vi "FPGAController_v4.2.vi"() -> ()   [LabVIEW 2015]
uses:
  <vilib>/Utility/miscctls.llb/LVPointTypeDef.ctl
  <vilib>/FPGAPlugInAG/PXI-7954R/niLvFpga_Open_PXI-7954R.vi
  <userlib>/_OpenG.lib/file/file.llb/Strip Path Extension - Path__ogtk.vi
  <userlib>/_OpenG.lib/comparison/comparison.llb/DBL Changed__ogtk.vi
  <vilib>/Utility/error.llb/Error Cluster From Error Code.vi
  <vilib>/rvi/errors/niLvFpgaAdjustHostInterfaceError.vi
  <vilib>/addons/database/Connection.llb/Conn Execute.vi
  <vilib>/addons/database/Recordset.llb/Rec Fetch Recordset Data (R).vi
  <vilib>/addons/database/Recordset.llb/Rec Destroy - Connection.vi
  <vilib>/FPGAPlugInAG/PXI-7954R/niLvFpga_Close_PXI-7954R.vi
  <vilib>/rvi/interface/nirviOpenFPGA/nirviOpenFPGA.xnode
  FPGA Bitfiles/correlationwithf_FPGATarget_FPGAcode60214_dpdmgs7o1BA.lvbitx
  <vilib>/rvi/interface/nirviMethod/nirviMethod.xnode
  <vilib>/FPGA/interface/niFpgaViExecutionMode.ctl
  <vilib>/rvi/interface/nirviReadWriteControl/nirviReadWriteControl.xnode
  <vilib>/addons/database/_DB Variant To Data/Database Variant To Data.xnode
  <vilib>/rvi/interface/nirviCloseFPGA/nirviCloseFPGA.xnode
  <vilib>/addons/database/NI_Database_API.lvlib
  NiFpgaLv.dll
panel:
  in  "Tab Control":enum32{"Auto Threshold", "Manual Threshold"}(tab)
  in  "Refresh PSU":bool=TRUE
  in  "Auto Threshold":bool
  in  "Update All":bool
  in  "Raise Threshold":bool
  in  "Lower Threshold":bool
  in  "Threshold 1":bool
  in  "Threshold 2":bool
  in  "Threshold 3":bool
  in  "Threshold 4":bool
  in  "Threshold 5":bool
  in  "Threshold 6":bool
  in  "Threshold 7":bool
  in  "Update By":i32
  out "Time Betwee Shots":dbl
  out "Del Armed":bool
  out "Update Threshold":bool
  in  "Min. Time\nBetween Shots (s)":dbl
  in  "Rate Limiting":bool
  out "Armed":bool
  in  "Add Delay":bool
  in  "Delay Name":string
  in  "Delay Value":dbl=3.0 min=0.0
  in  "Delay Ring":dbl(ring)=3.15039 items=["Custom"]
  in  "Rearm Trigger":bool
  in  "One Shot Mode":bool
  out "Last Update:":timestamp
  out "Updating FPGA":bool
  out "Sensitivity":dbl
  out "error out":errorcluster
  out "Low Mass Limit":fxp<+,31,17>
  out "High Mass Limit":fxp<+,31,17>
  out "stopping":bool
  out "Peletron (MV)":dbl=2.0
  out "High Mass (kg)":dbl=inf
  out "Low Mass (kg)":dbl
  out "High Charge Limit":i16
  out "Low Charge Limit":i16
  out "High velocity count":i32=210
  out "Low velocity count":i32=21000
  in  "stop":bool
  in  "Peak-Threshold Factor":dbl=2.0
  out "Low Charge Limit (fC)":dbl
  out "High Charge Limit (fC)":dbl=100.0
  out "High Velocity":dbl=100000.0
  out "Low Velocity":dbl=1000.0
  out "Filter 7 Peak":i32=7483
  out "Filter 6 Peak":i32=9863
  out "Filter 5 Peak":i32=13910
  out "Filter 4 Peak":i32=18191
  out "Filter 3 Peak":i32=46254
  out "Filter 2 Peak":i32=120664
  out "Filter 1 Peak":i32=295996
  in  "Filter7 Threshold":i32=-21165
  in  "Filter6 Threshold":i32=-29358
  in  "Filter5 Threshold":i32=-41730
  in  "Filter4 Threshold":i32=-54306
  in  "Filter3 Threshold":i32=-138762
  in  "Filter2 Threshold":i32=-361992
  in  "Filter1 Threshold":i32=-887988
  in  "Zero Peak Values":bool
  in  "Assign Threshold":bool
  in  "Run Mode":bool
  # "Settings"
  # "Dubugging"
  # "Independent Variable"
  # "Low Vel."
  # "High Vel."
  # "Low Q (fC)"
  # "High Q (fC)"
  # "Plate Control While Loop Counter"
  # "Low Mass (kg)"
  # "High Mass (kg)"
  # "Sens. (V/pC)"
  # "Peletron (MV)"
  # "Current Value of Running Average"
  # "Peak Threshold Factor"
  # "Delay Trigger"
  # "Dist. from 2nd Det. (m)"
  # "Name"
  # "Peak Values"
  # "Peak 1"
  # "Peak 2"
  # "Peak 3"
  # "Peak 4"
  # "Peak 5"
  # "Peak 6"
  # "Peak 7"
  # "Thresholds"
  # "Threshold 1"
  # "Threshold 2"
  # "Threshold 3"
  # "Threshold 4"
  # "Threshold 5"
  # "Threshold 6"
  # "Threshold 7"
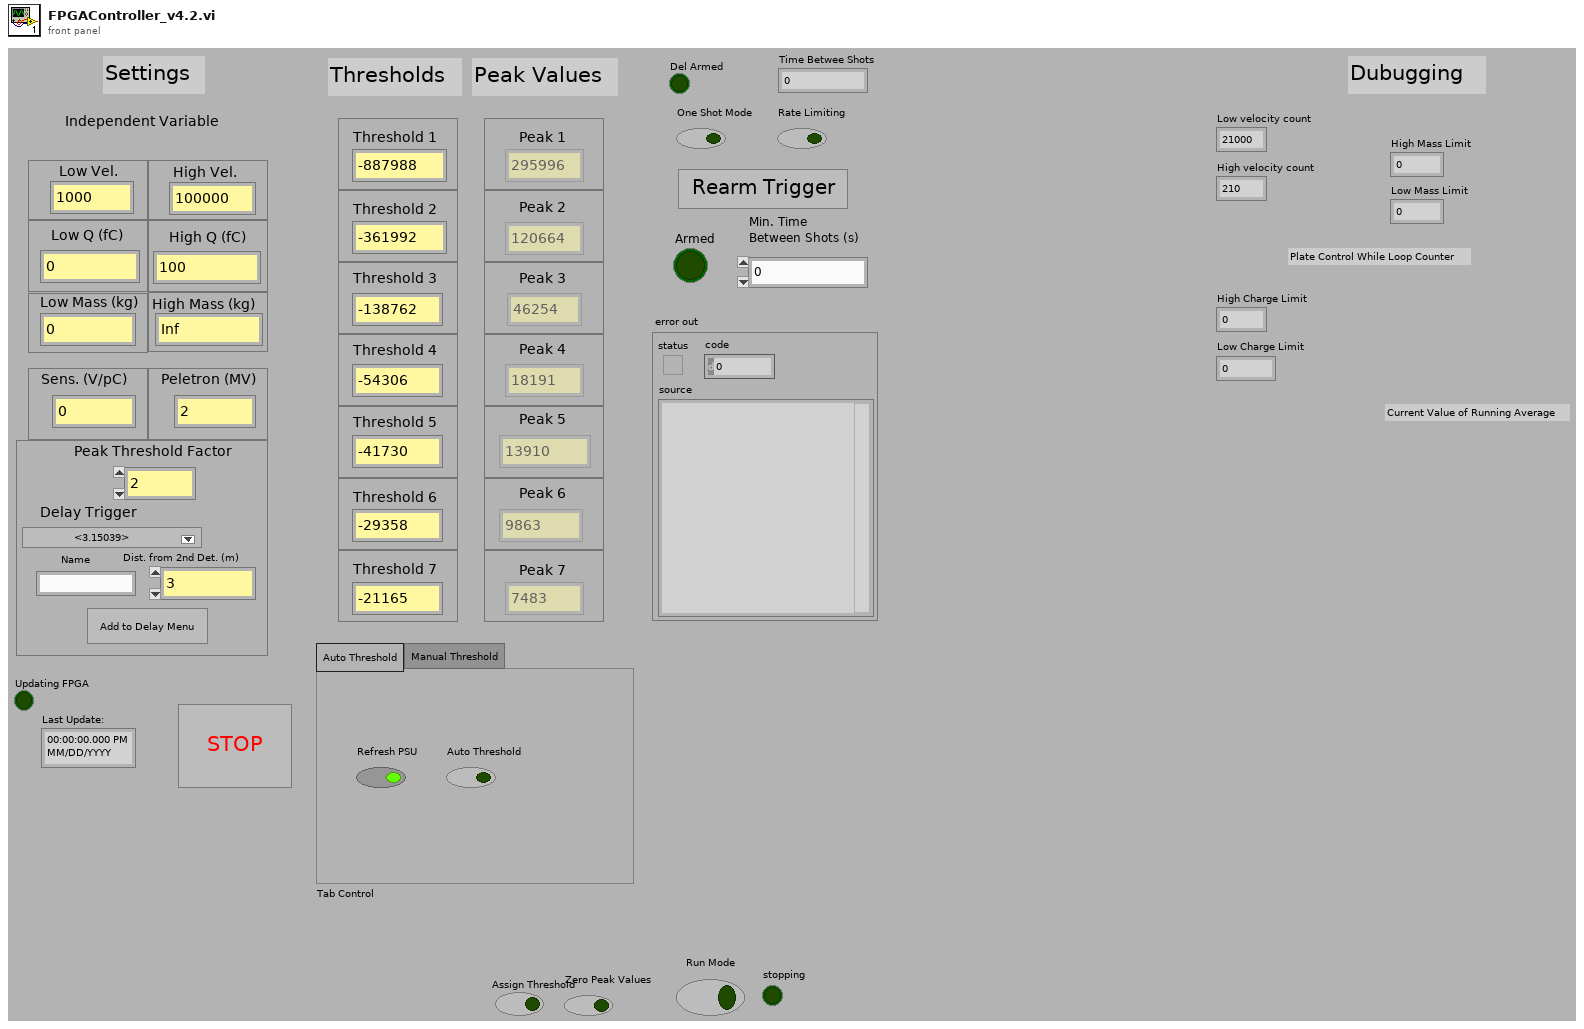
[diagram p1: front panel]
types:
  T1 = typedef "LVPointTypeDef.ctl" = cluster{"Horizontal":i16, "Vertical":i16}
  T2 = enum8{"Enabled", "Disabled", "Disabled and Grayed Out"}
  T3 = typedef "NI_Database_API.lvlib/Conn ObjectReference.ctl" = refnum<k1>
  T4 = typedef "NI_Database_API.lvlib/Rec ObjectReference.ctl" = refnum<k1>
  T5 = cluster{"Filter 1 Peak":i32, "Filter 2 Peak":i32, "Filter 3 Peak":i32, "Filter 4 Peak":i32, "Filter 5 Peak":i32, "Filter 6 Peak":i32, "Filter 7 Peak":i32}
  T6 = typedef "LVStringsAndValuesArrayTypeDef_DBL.ctl" = cluster{"String":string, "Value":dbl}[]
  T7 = cluster{"Numeric":dbl, "Numeric":dbl, "Numeric":dbl, "Numeric":dbl, "Numeric":dbl, "Numeric":dbl, "Sensitivity":dbl, dbl, "Value":dbl, fxp<+,16,7>, bool}
  T8 = cluster{"Low Velocity Count":i32, "High Velocity Count":i32, "Low Charge Limit (ADC ticks)":i16, "High Charge Limit (ADC ticks)":i16, "Low Mass (ADC*cycle^2)":i64, "High Mass (ADC*cycle^2)":i64, "Mult":fxp<+,16,7>, "Mult Use?":bool}
  T9 = cluster{"Filter 1 Detector 3 Correlation":i32, "Filter 2 Detector 3 Correlation":i32, "Filter 3 Detector 3 Correlation":i32, "Filter 4 Detector 3 Correlation":i32, "Filter 5 Detector 3 Correlation":i32, "Filter 6 Detector 3 Correlation":i32, "Filter 7 Detector 3 Correlation":i32}
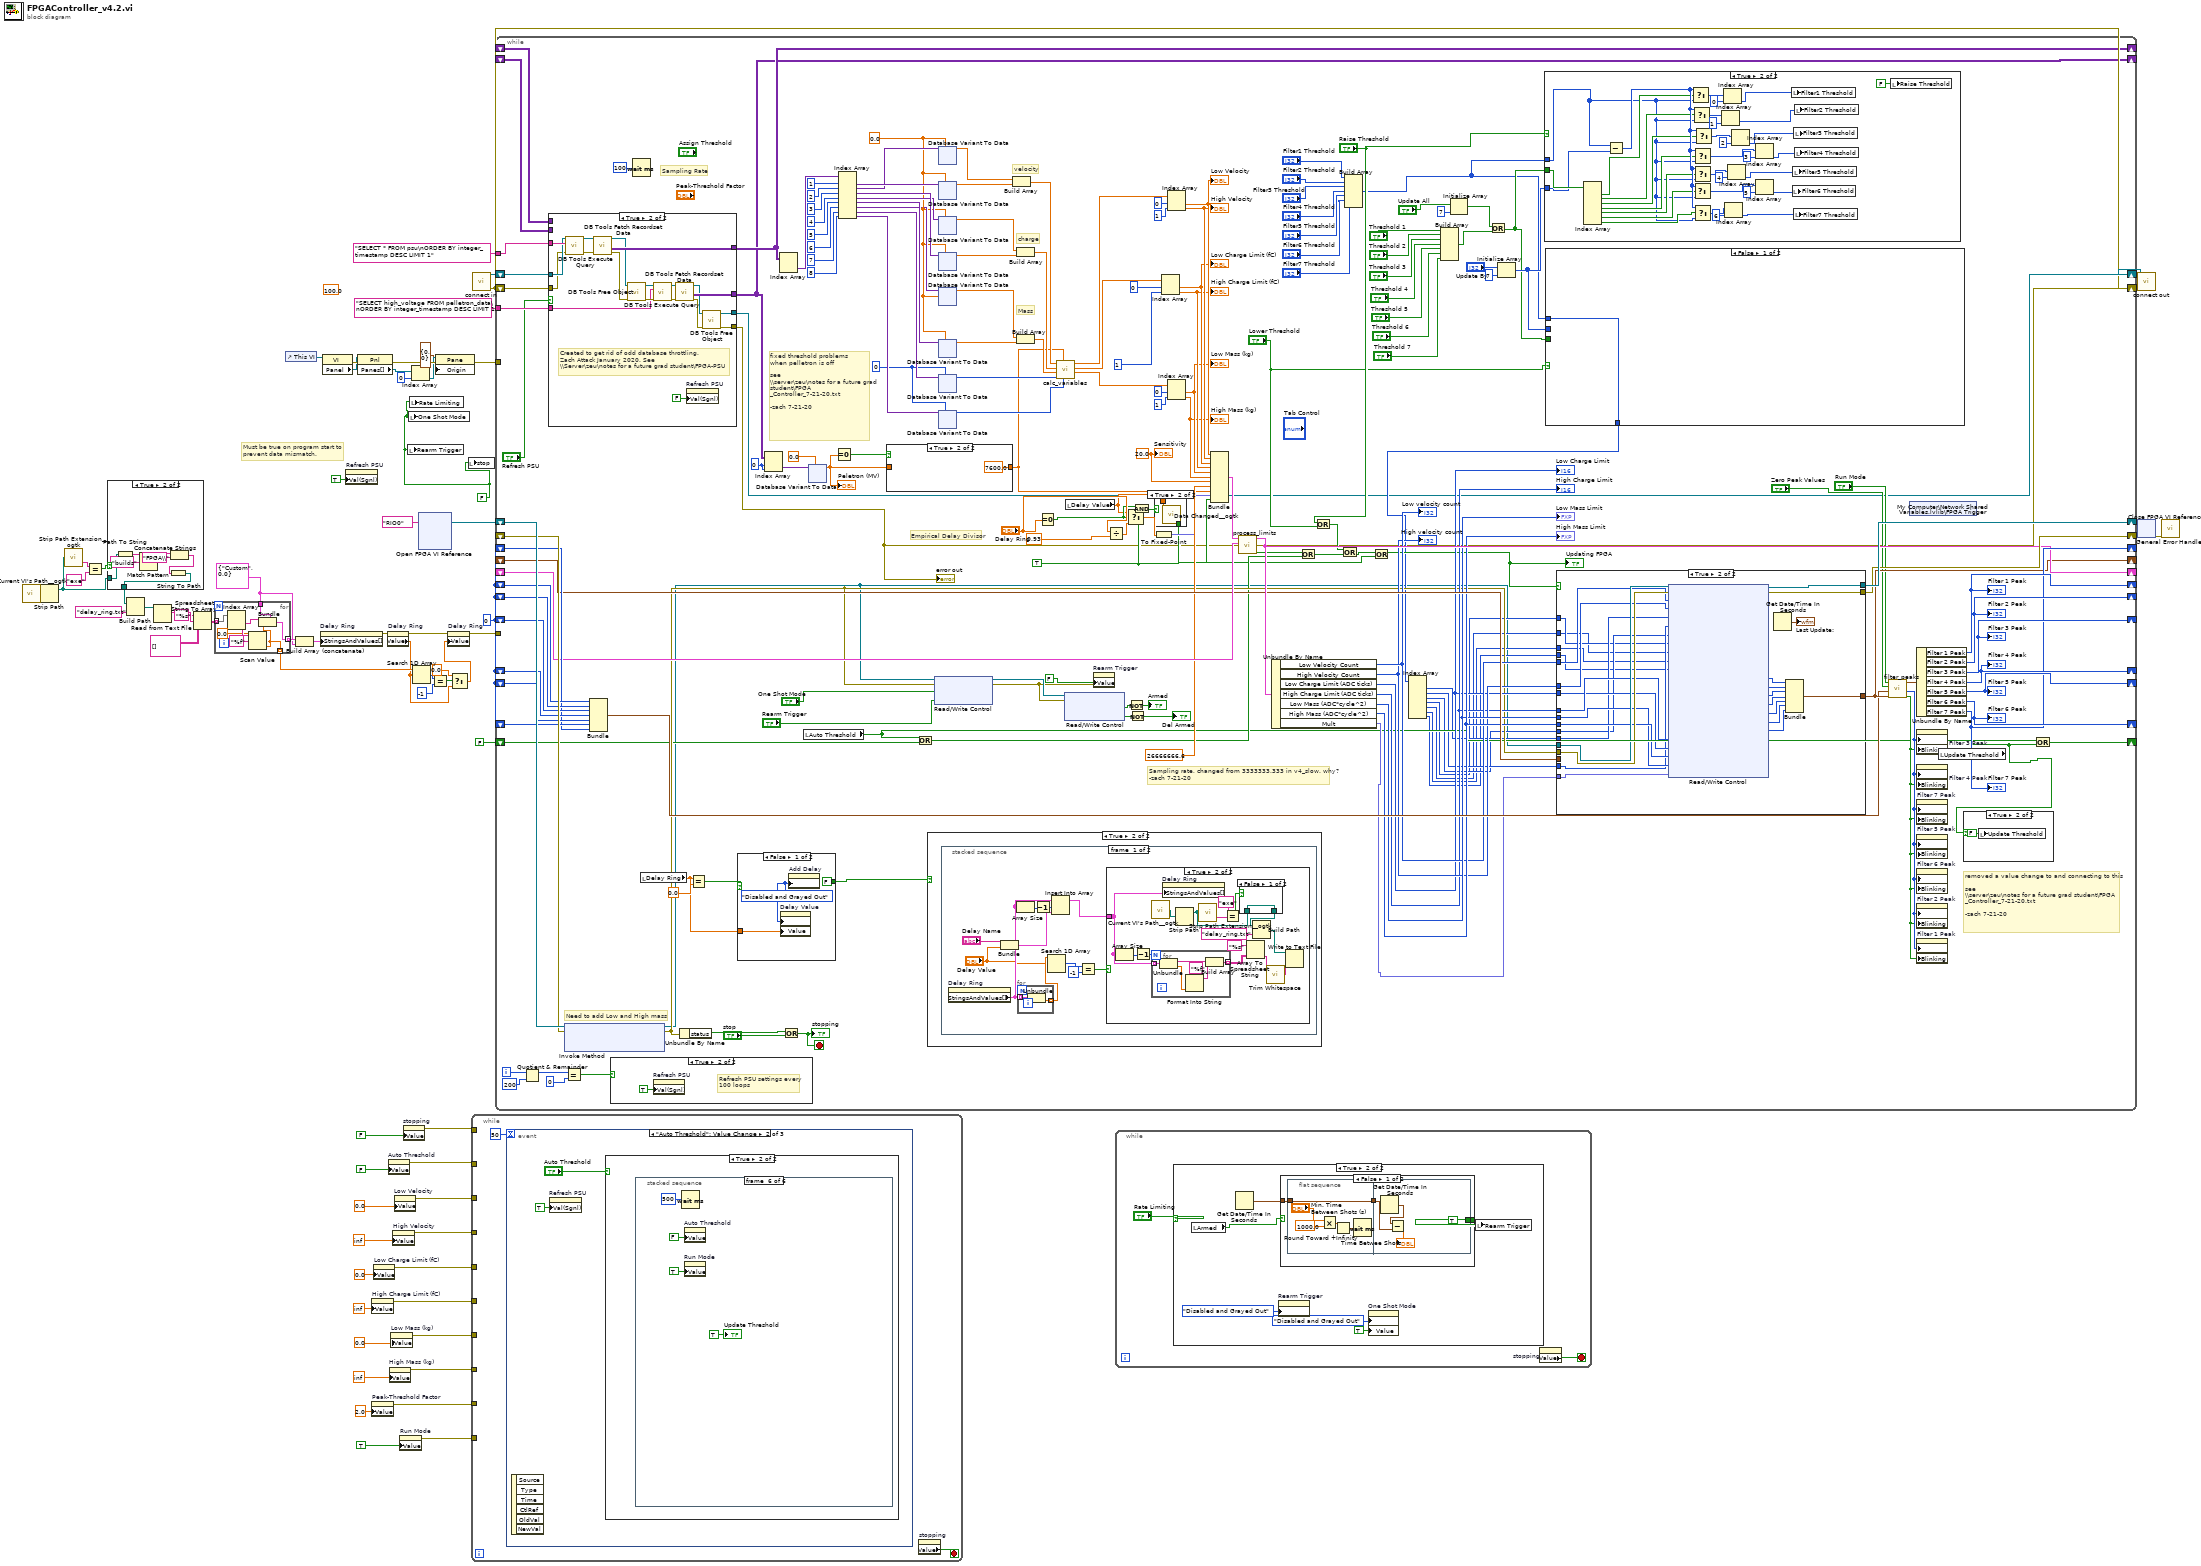
[diagram p0: block diagram]
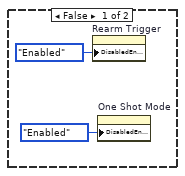
[diagram p3: hidden frame]
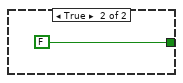
[diagram p4: hidden frame]
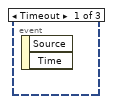
[diagram p5: hidden frame]
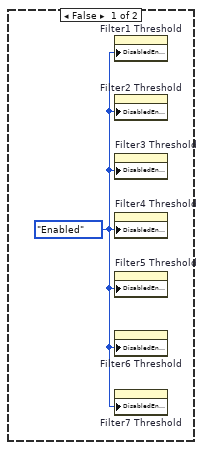
[diagram p6: hidden frame]
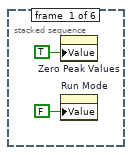
[diagram p7: hidden frame]
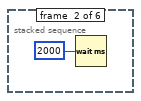
[diagram p8: hidden frame]
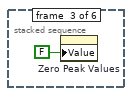
[diagram p9: hidden frame]
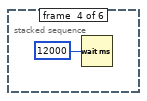
[diagram p10: hidden frame]
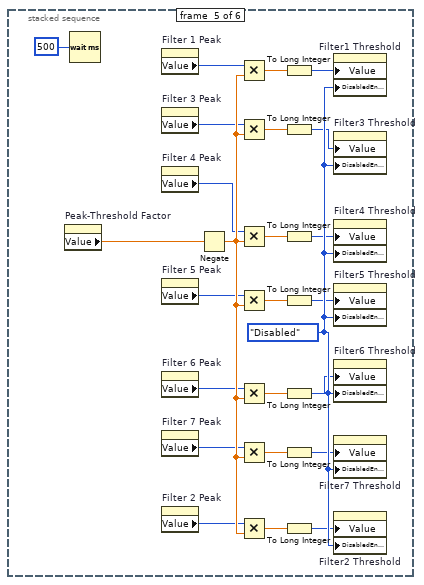
[diagram p11: hidden frame]
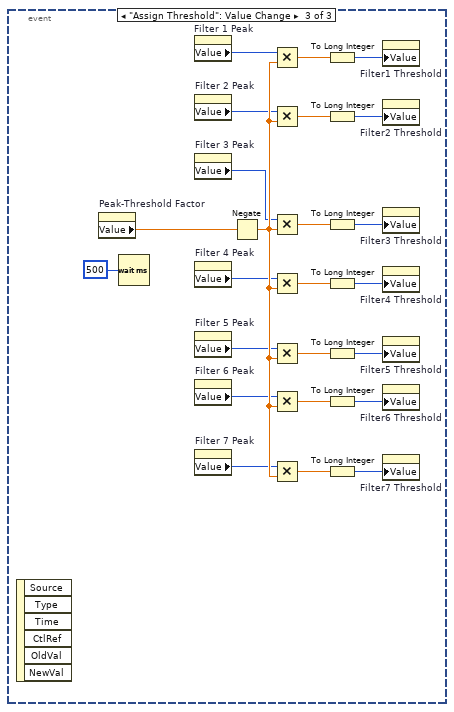
[diagram p12: hidden frame]
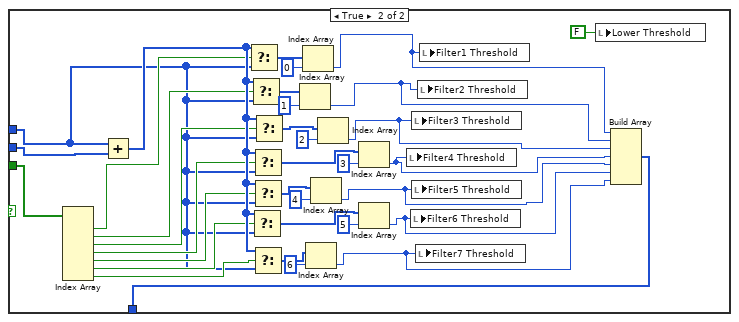
[diagram p16: hidden frame]
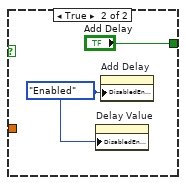
[diagram p20: hidden frame]
diagram:
  (unwired) 100.0 ("Update By")
  w19 = cluster{"String":string, "Value":dbl} {"String"="Custom", "Value"=0.0}
  w29 = FALSE
  w67 = 0
  # "Must be true on program start to\nprevent data mismatch."
  n1 = call <userlib>:"Current VI's Path__ogtk.vi"() -> ("Current VI's Path (+ Relative)"=w28:path)  [unwired: 1 in]
  n2 = Strip Path(path=w28) -> (stripped path=w14:path)  [unwired: 1 out]
  n3 = call-poly <userlib>:"Strip Path Extension__ogtk.vi"("path"=w14) -> ("extension"=w18:string)  [unwired: 1 out]
  n4 = Equal?(x=w18, y="exe") -> (x = y?=w15:bool)
  n5 = case shown="True" w15 {
    tunnel: w14 -> [w69 w76]
    tunnel: [w69 w70] -> w13
    frame False {
    }
    frame True {
      n6 = Path To String(path=w76) -> (string=w75:string)
      n7 = Match Pattern(string=w75, regular expression="builds") -> (before substring=w73:string)  [unwired: 1 in, 3 out]
      n8 = Concatenate Strings(w73, "FPGA\\" ("string")) -> (w71:string)
      n9 = String To Path(string=w71) -> (path=w70:path)
    }
  }
  n10 = Build Path(base path=w13, name or relative path="delay_ring.txt") -> (appended path=w16:path)
  n11 = Read from Text File(file (use dialog)=w16) -> (text=w26:string)  [unwired: 3 in, 3 out]
  n12 = Spreadsheet String To Array(format string="%s", spreadsheet string=w26, array type (2D Dbl)=string[][] []) -> (array=w23:string[][])  [unwired: 1 in]
  n13 = for {
    tunnel: w23 -> [w84] mode=indexing
    tunnel: w19 -> [w82]
    tunnel: [w78] -> w20 mode=indexing
    tunnel: [w77] -> w12 mode=indexing
    n14 = Index Array(array=w84) -> (element #1=w83:string, element #2=w81:string)  [unwired: 2 in]
    n15 = Scan Value(string=w81, format string="%f", default (0 dbl)=0.0) -> (value=w77:dbl)  [unwired: 1 out]
    n16 = Bundle(cluster=w82, "String"=w83, "Value"=w77) -> (w78:cluster{"String":string, "Value":dbl})
  }
  n17 = control-ref of="This VI"() -> (w40:refnum<vi>)
  n18 = Build Array (concatenate)(w20, w19) -> (w22:cluster{"String":string, "Value":dbl}[])
  n19 = property on="Delay Ring" class="Ring (strict)"("StringsAndValues[]"=w22) -> (error out=w21:errorcluster)  [unwired: 2 in, 1 out]
  n20 = property class="VI"(reference=w40) -> (error out=w39:errorcluster, "Panel"=w38:refnum<vi>)  [unwired: 1 in, 1 out]
  n21 = property on="Refresh PSU" class="Bool (strict)"("Val(Sgnl)"=TRUE ("Value (Signaling)")) -> ()  [unwired: 2 in, 2 out]
  n22 = property class="Pnl"(reference=w38, error in=w39) -> (error out=w37:errorcluster, "Panes[]"=w36:refnum<vi>[])  [unwired: 1 out]
  n23 = property on="High Charge Limit (fC)" class="DigNum (strict)"("Value"=inf ("High Charge Limit (fC)")) -> (error out=w54:errorcluster)  [unwired: 2 in, 1 out]
  n24 = property on="Peak-Threshold Factor" class="DigNum (strict)"("Value"=2.0 ("Peak-Threshold Factor")) -> (error out=w48:errorcluster)  [unwired: 2 in, 1 out]
  n25 = property on="Low Charge Limit (fC)" class="DigNum (strict)"("Value"=0.0 ("Low Charge Limit (fC)")) -> (error out=w56:errorcluster)  [unwired: 2 in, 1 out]
  n26 = property on="Delay Ring" class="Ring (strict)"(error in=w21) -> (error out=w11:errorcluster, "Value"=w5:dbl)  [unwired: 1 in, 1 out]
  n27 = property on="Auto Threshold" class="Bool (strict)"("Value"=FALSE ("Auto Threshold")) -> (error out=w62:errorcluster)  [unwired: 2 in, 1 out]
  n28 = property on="High Mass (kg)" class="DigNum (strict)"("Value"=inf ("High Mass (kg)")) -> (error out=w50:errorcluster)  [unwired: 2 in, 1 out]
  n29 = property on="Low Mass (kg)" class="DigNum (strict)"("Value"=0.0 ("Low Mass (kg)")) -> (error out=w52:errorcluster)  [unwired: 2 in, 1 out]
  n30 = property on="High Velocity" class="DigNum (strict)"("Value"=inf ("High Velocity")) -> (error out=w58:errorcluster)  [unwired: 2 in, 1 out]
  n31 = property on="Low Velocity" class="DigNum (strict)"("Value"=0.0 ("Low Velocity")) -> (error out=w60:errorcluster)  [unwired: 2 in, 1 out]
  n32 = property on="Run Mode" class="Bool (strict)"("Value"=TRUE ("Run Mode")) -> (error out=w46:errorcluster)  [unwired: 2 in, 1 out]
  n33 = property on="stopping" class="Bool (strict)"("Value"=FALSE ("stopping")) -> (error out=w64:errorcluster)  [unwired: 2 in, 1 out]
  n34 = local write "Rearm Trigger"(w29) -> ()
  n35 = local write "One Shot Mode"(w29) -> ()
  n36 = local write "Rate Limiting"(w29) -> ()
  n37 = Index Array(array=w36, index=0) -> (element=w34:refnum<vi>)
  n38 = Search 1D Array(1D array=w12, element=w5) -> (index of element=w9:i32)  [unwired: 1 in]
  n39 = xnode "Open FPGA VI Reference"("resource name"=tag "RIO0") -> ("FPGA VI Reference Out"=w31:refnum<k20>)  [unwired: 1 in, 1 out]
  n40 = Equal?(x=w9, y=-1) -> (x = y?=w7:bool)
  n41 = property class="Pane"(reference=w34, error in=w37, "Origin"=T1 {"Horizontal"=0, "Vertical"=0}) -> (error out=w32:errorcluster)  [unwired: 1 out]
  n42 = Select(t=0.0, s=w7, f=w5) -> (s? t:f=w6:dbl)
  n43 = property on="Delay Ring" class="Ring (strict)"(error in=w11, "Value"=w6) -> (error out=w10:errorcluster)  [unwired: 1 in, 1 out]
  n44 = local write "stop"(w29) -> ()
  n45 = while {
    tunnel: w64 -> [_]
    tunnel: w62 -> [_]
    tunnel: w60 -> [_]
    tunnel: w58 -> [_]
    tunnel: w56 -> [_]
    tunnel: w54 -> [_]
    tunnel: w52 -> [_]
    tunnel: w50 -> [_]
    tunnel: w48 -> [_]
    tunnel: w46 -> [_]
    stop <- w86 stop-if-true
    n46 = event shown="[1] \"Auto Threshold\": Value Change" {
      selector: _ -> [_ _ _]
      dyn-events: _ -> [_ _ _]
      timeout: 50 -> [_ _ _]
      event Timeout {
        n47 = event-data() -> ()  [unwired: 1 in, 2 out]
      }
      event "Auto Threshold": Value Change {
        n48 = event-data() -> ()  [unwired: 1 in, 6 out]
        n49 = property on="Refresh PSU" class="Bool (strict)"("Val(Sgnl)"=TRUE ("Value (Signaling)")) -> ()  [unwired: 2 in, 2 out]
        n50 = case shown="True" "Auto Threshold" {
          frame False {
            w89 = T2."Enabled" ("Disabled")
            n51 = property on="Filter1 Threshold" class="DigNum (strict)"("DisabledEnum"=w89) -> ()  [unwired: 2 in, 2 out]
            n52 = property on="Filter2 Threshold" class="DigNum (strict)"("DisabledEnum"=w89) -> ()  [unwired: 2 in, 2 out]
            n53 = property on="Filter3 Threshold" class="DigNum (strict)"("DisabledEnum"=w89) -> ()  [unwired: 2 in, 2 out]
            n54 = property on="Filter4 Threshold" class="DigNum (strict)"("DisabledEnum"=w89) -> ()  [unwired: 2 in, 2 out]
            n55 = property on="Filter5 Threshold" class="DigNum (strict)"("DisabledEnum"=w89) -> ()  [unwired: 2 in, 2 out]
            n56 = property on="Filter6 Threshold" class="DigNum (strict)"("DisabledEnum"=w89) -> ()  [unwired: 2 in, 2 out]
            n57 = property on="Filter7 Threshold" class="DigNum (strict)"("DisabledEnum"=w89) -> ()  [unwired: 2 in, 2 out]
          }
          frame True {
            n58 = stacked-sequence {
              frame #0 {
                n59 = property on="Zero Peak Values" class="Bool (strict)"("Value"=TRUE ("Zero Peak Values")) -> ()  [unwired: 2 in, 2 out]
                n60 = property on="Run Mode" class="Bool (strict)"("Value"=FALSE ("Run Mode")) -> ()  [unwired: 2 in, 2 out]
              }
              frame #1 {
                n61 = Wait (ms)(milliseconds to wait=u32 2000) -> ()  [unwired: 1 out]
              }
              frame #2 {
                n62 = property on="Zero Peak Values" class="Bool (strict)"("Value"=FALSE ("Zero Peak Values")) -> ()  [unwired: 2 in, 2 out]
              }
              frame #3 {
                n63 = Wait (ms)(milliseconds to wait=u32 12000) -> ()  [unwired: 1 out]
              }
              frame #4 {
                w119 = T2."Disabled" ("Disabled")
                n64 = property on="Peak-Threshold Factor" class="DigNum (strict)"() -> ("Value"=w104:dbl)  [unwired: 2 in, 2 out]
                n65 = Wait (ms)(milliseconds to wait=u32 500) -> ()  [unwired: 1 out]
                n66 = property on="Filter 1 Peak" class="DigNum (strict)"() -> ("Value"=w102:i32)  [unwired: 2 in, 2 out]
                n67 = property on="Filter 3 Peak" class="DigNum (strict)"() -> ("Value"=w100:i32)  [unwired: 2 in, 2 out]
                n68 = property on="Filter 4 Peak" class="DigNum (strict)"() -> ("Value"=w99:i32)  [unwired: 2 in, 2 out]
                n69 = property on="Filter 5 Peak" class="DigNum (strict)"() -> ("Value"=w98:i32)  [unwired: 2 in, 2 out]
                n70 = property on="Filter 6 Peak" class="DigNum (strict)"() -> ("Value"=w97:i32)  [unwired: 2 in, 2 out]
                n71 = property on="Filter 7 Peak" class="DigNum (strict)"() -> ("Value"=w96:i32)  [unwired: 2 in, 2 out]
                n72 = property on="Filter 2 Peak" class="DigNum (strict)"() -> ("Value"=w101:i32)  [unwired: 2 in, 2 out]
                n73 = Negate(x=w104) -> (-x=w103:dbl)
                n74 = Multiply(x=w102, y=w103) -> (x*y=w118:dbl)
                n75 = Multiply(x=w100, y=w103) -> (x*y=w114:dbl)
                n76 = Multiply(x=w99, y=w103) -> (x*y=w112:dbl)
                n77 = Multiply(x=w98, y=w103) -> (x*y=w110:dbl)
                n78 = Multiply(x=w97, y=w103) -> (x*y=w108:dbl)
                n79 = Multiply(x=w96, y=w103) -> (x*y=w106:dbl)
                n80 = Multiply(x=w101, y=w103) -> (x*y=w116:dbl)
                n81 = To Long Integer(number=w118) -> (32bit integer=w117:i32)
                n82 = To Long Integer(number=w114) -> (32bit integer=w113:i32)
                n83 = To Long Integer(number=w112) -> (32bit integer=w111:i32)
                n84 = To Long Integer(number=w110) -> (32bit integer=w109:i32)
                n85 = To Long Integer(number=w108) -> (32bit integer=w107:i32)
                n86 = To Long Integer(number=w106) -> (32bit integer=w105:i32)
                n87 = To Long Integer(number=w116) -> (32bit integer=w115:i32)
                n88 = property on="Filter1 Threshold" class="DigNum (strict)"("Value"=w117, "DisabledEnum"=w119) -> ()  [unwired: 2 in, 2 out]
                n89 = property on="Filter3 Threshold" class="DigNum (strict)"("Value"=w113, "DisabledEnum"=w119) -> ()  [unwired: 2 in, 2 out]
                n90 = property on="Filter4 Threshold" class="DigNum (strict)"("Value"=w111, "DisabledEnum"=w119) -> ()  [unwired: 2 in, 2 out]
                n91 = property on="Filter5 Threshold" class="DigNum (strict)"("Value"=w109, "DisabledEnum"=w119) -> ()  [unwired: 2 in, 2 out]
                n92 = property on="Filter6 Threshold" class="DigNum (strict)"("Value"=w107, "DisabledEnum"=w119) -> ()  [unwired: 2 in, 2 out]
                n93 = property on="Filter7 Threshold" class="DigNum (strict)"("Value"=w105, "DisabledEnum"=w119) -> ()  [unwired: 2 in, 2 out]
                n94 = property on="Filter2 Threshold" class="DigNum (strict)"("Value"=w115, "DisabledEnum"=w119) -> ()  [unwired: 2 in, 2 out]
              }
              frame #5 {
                n95 = Wait (ms)(milliseconds to wait=u32 500) -> ()  [unwired: 1 out]
                n96 = property on="Auto Threshold" class="Bool (strict)"("Value"=FALSE ("Auto Threshold")) -> ()  [unwired: 2 in, 2 out]
                n97 = property on="Run Mode" class="Bool (strict)"("Value"=TRUE ("Run Mode")) -> ()  [unwired: 2 in, 2 out]
                "Update Threshold" <- TRUE ("Update Threshold")
              }
            }
          }
        }
      }
      event "Assign Threshold": Value Change {
        n98 = event-data() -> ()  [unwired: 1 in, 6 out]
        n99 = property on="Peak-Threshold Factor" class="DigNum (strict)"() -> ("Value"=w138:dbl)  [unwired: 2 in, 2 out]
        n100 = Wait (ms)(milliseconds to wait=u32 500) -> ()  [unwired: 1 out]
        n101 = property on="Filter 1 Peak" class="DigNum (strict)"() -> ("Value"=w137:i32)  [unwired: 2 in, 2 out]
        n102 = property on="Filter 2 Peak" class="DigNum (strict)"() -> ("Value"=w136:i32)  [unwired: 2 in, 2 out]
        n103 = property on="Filter 3 Peak" class="DigNum (strict)"() -> ("Value"=w135:i32)  [unwired: 2 in, 2 out]
        n104 = property on="Filter 4 Peak" class="DigNum (strict)"() -> ("Value"=w134:i32)  [unwired: 2 in, 2 out]
        n105 = property on="Filter 5 Peak" class="DigNum (strict)"() -> ("Value"=w133:i32)  [unwired: 2 in, 2 out]
        n106 = property on="Filter 6 Peak" class="DigNum (strict)"() -> ("Value"=w132:i32)  [unwired: 2 in, 2 out]
        n107 = property on="Filter 7 Peak" class="DigNum (strict)"() -> ("Value"=w131:i32)  [unwired: 2 in, 2 out]
        n108 = Negate(x=w138) -> (-x=w140:dbl)
        n109 = Multiply(x=w137, y=w140) -> (x*y=w147:dbl)
        n110 = Multiply(x=w136, y=w140) -> (x*y=w145:dbl)
        n111 = Multiply(x=w135, y=w140) -> (x*y=w144:dbl)
        n112 = Multiply(x=w134, y=w140) -> (x*y=w143:dbl)
        n113 = Multiply(x=w133, y=w140) -> (x*y=w142:dbl)
        n114 = Multiply(x=w132, y=w140) -> (x*y=w141:dbl)
        n115 = Multiply(x=w131, y=w140) -> (x*y=w146:dbl)
        n116 = To Long Integer(number=w147) -> (32bit integer=w130:i32)
        n117 = To Long Integer(number=w145) -> (32bit integer=w129:i32)
        n118 = To Long Integer(number=w144) -> (32bit integer=w128:i32)
        n119 = To Long Integer(number=w143) -> (32bit integer=w127:i32)
        n120 = To Long Integer(number=w142) -> (32bit integer=w126:i32)
        n121 = To Long Integer(number=w141) -> (32bit integer=w125:i32)
        n122 = To Long Integer(number=w146) -> (32bit integer=w124:i32)
        n123 = property on="Filter1 Threshold" class="DigNum (strict)"("Value"=w130) -> ()  [unwired: 2 in, 2 out]
        n124 = property on="Filter2 Threshold" class="DigNum (strict)"("Value"=w129) -> ()  [unwired: 2 in, 2 out]
        n125 = property on="Filter3 Threshold" class="DigNum (strict)"("Value"=w128) -> ()  [unwired: 2 in, 2 out]
        n126 = property on="Filter4 Threshold" class="DigNum (strict)"("Value"=w127) -> ()  [unwired: 2 in, 2 out]
        n127 = property on="Filter5 Threshold" class="DigNum (strict)"("Value"=w126) -> ()  [unwired: 2 in, 2 out]
        n128 = property on="Filter6 Threshold" class="DigNum (strict)"("Value"=w125) -> ()  [unwired: 2 in, 2 out]
        n129 = property on="Filter7 Threshold" class="DigNum (strict)"("Value"=w124) -> ()  [unwired: 2 in, 2 out]
      }
    }
    n130 = property on="stopping" class="Bool (strict)"() -> ("Value"=w86:bool)  [unwired: 2 in, 2 out]
  }
  n131 = call "connect in.vi"() -> ("error out"=w41:errorcluster, "Database Connection"=w42:T3)  [unwired: 7 in, 1 out]
  n132 = while {
    shift-right: [w320] -> w66
    shift-left: w31 -> [w324]
    shift-right: [w319] -> w65
    shift-left: _ -> [w323]
    shift-right: [w315] -> _
    shift-left: w67 -> [w308]
    shift-right: [w314] -> _
    shift-left: w67 -> [w307]
    shift-right: [w313] -> _
    shift-left: w67 -> [w306]
    shift-right: [w312] -> _
    shift-left: w67 -> [w305]
    shift-right: [w311] -> _
    shift-left: w67 -> [w304]
    shift-right: [w317] -> _
    shift-left: w67 -> [w310]
    shift-right: [w316] -> _
    shift-left: w67 -> [w309]
    tunnel: "SELECT * FROM psu\nORDER BY integer_timestamp DESC LIMIT 1" ("SQL query") -> [w169]
    shift-right: [w165] -> w43
    shift-left: w42 -> [w168]
    shift-right: [w164] -> _
    shift-left: w41 -> [w167]
    shift-right: [w303] -> _
    shift-left: _ -> [w302]
    shift-right: [w300] -> _
    shift-left: _ -> [w301]
    tunnel: w32 -> [_]
    tunnel: w10 -> [_]
    shift-right: [w219] -> _
    shift-left: FALSE -> [w222]
    tunnel: "SELECT high_voltage FROM pelletron_data\nORDER BY integer_timestamp DESC LIMIT 1" ("SQL query") -> [w166]
    shift-right: [w163] -> _
    shift-left: _ -> [w162]
    shift-right: [w161] -> _
    shift-left: _ -> [w160]
    i -> [w158]
    stop <- w318 stop-if-true
    w151 = 20.0 ("Sensitivity")
    w191 = TRUE
    w266 = 0 ("index (row)")
    w267 = i8 0
    w268 = 0.0
    # "fixed threshold problems\nwhen pelletron is off\n\nsee \n\\\\server\\zeu\\notes for a future grad student\\FPGA\n_Controller_7-21-20.txt\n\n-zach 7-21-20"
    # "Sampling rate, changed from 3333333.333 in v4_slow. why?\n-zach 7-21-20"
    # "removed a value change to and connecting to this\n\nsee \n\\\\server\\zeu\\notes for a future grad student\\FPGA\n_Controller_7-21-20.txt\n\n-zach 7-21-20"
    # "charge"
    # "Empirical Delay Divisor"
    # "Mass"
    # "velocity"
    # "Sampling Rate"
    # "Need to add Low and High mass"
    n133 = Quotient & Remainder(x=w158, y=200) -> (x-y*floor(x/y)=w156:i32)  [unwired: 1 out]
    n134 = case shown="True" "Refresh PSU" {
      tunnel: [w329 w348] -> w163
      tunnel: w169 -> [_ w347]
      tunnel: w168 -> [w331 w346]
      tunnel: w167 -> [w330 w345]
      tunnel: w166 -> [_ w338]
      tunnel: [w328 w337] -> w161
      tunnel: [w331 w334] -> w165
      tunnel: [w330 w333] -> w164
      tunnel: w162 -> [w329 _]
      tunnel: w160 -> [w328 _]
      frame False {
      }
      frame True {
        # "Created to get rid of odd database throttling.\nZach Attack January 2020. See \n\\\\Server\\zeu\\notes for a future grad student\\FPGA-PSU"
        n135 = call-poly <vilib>:"DB Tools Execute Query.vi"("error in (no error)"=w345, "SQL query"=w347, "connection reference"=w346) -> ("error out"=w349:errorcluster, "recordset reference"=w350:T4)  [unwired: 5 in]
        n136 = call-poly <vilib>:"DB Tools Fetch Recordset Data.vi"("error in (no error)"=w349, "recordset reference"=w350) -> ("error out"=w339:errorcluster, "recordset data"=w348:variant[][], "recordset reference out"=w342:T4)  [unwired: 3 in]
        n137 = call-poly <vilib>:"DB Tools Free Object.vi"("error in (no error)"=w339, "recordset reference"=w342) -> ("error out"=w340:errorcluster, "connection reference"=w341:T3)  [unwired: 8 in]
        n138 = call-poly <vilib>:"DB Tools Execute Query.vi"("error in (no error)"=w340, "SQL query"=w338, "connection reference"=w341) -> ("error out"=w344:errorcluster, "recordset reference"=w343:T4)  [unwired: 5 in]
        n139 = call-poly <vilib>:"DB Tools Fetch Recordset Data.vi"("error in (no error)"=w344, "recordset reference"=w343) -> ("error out"=w335:errorcluster, "recordset data"=w337:variant[][], "recordset reference out"=w336:T4)  [unwired: 3 in]
        n140 = property on="Refresh PSU" class="Bool (strict)"("Val(Sgnl)"=FALSE ("Value (Signaling)")) -> ()  [unwired: 2 in, 2 out]
        n141 = call-poly <vilib>:"DB Tools Free Object.vi"("error in (no error)"=w335, "recordset reference"=w336) -> ("error out"=w333:errorcluster, "connection reference"=w334:T3)  [unwired: 8 in]
      }
    }
    "error out" <- w164
    n142 = xnode "Invoke Method"("FPGA VI Reference In"=w324, "error in"=w323) -> ("FPGA VI Reference Out"=w152:refnum<k20>, "error out"=w238:errorcluster)  [unwired: 1 out]
    n143 = Equal?(x=w156, y=0) -> (x = y?=w154:bool)
    n144 = Bundle("Filter 1 Peak"=w310, "Filter 2 Peak"=w309, "Filter 3 Peak"=w308, "Filter 4 Peak"=w307, "Filter 5 Peak"=w306, "Filter 6 Peak"=w305, "Filter 7 Peak"=w304) -> (w296:T5)  [unwired: 1 in]
    n145 = case shown="True" w154 {
      frame False {
      }
      frame True {
        # "Refresh PSU settings every\n100 loops"
        n146 = property on="Refresh PSU" class="Bool (strict)"("Val(Sgnl)"=TRUE ("Value (Signaling)")) -> ()  [unwired: 2 in, 2 out]
      }
    }
    n147 = Wait (ms)(milliseconds to wait=u32 100) -> ()  [unwired: 1 out]
    n148 = local read "Delay Ring"() -> (w223:dbl)
    n149 = Unbundle By Name(w238) -> ("status"=w322:bool)
    n150 = Equal?(x=w223, y=0.0) -> (x = y?=w224:bool)
    n151 = case shown="False" w224 {
      tunnel: [FALSE ("Add Delay") "Add Delay"] -> w241
      tunnel: w223 -> [w424 _]
      frame False {
        w425 = T2."Disabled and Grayed Out" ("Disabled")
        n152 = property on="Delay Value" class="DigNum (strict)"("DisabledEnum"=w425, "Value"=w424) -> ()  [unwired: 2 in, 2 out]
        n153 = property on="Add Delay" class="Bool (strict)"("DisabledEnum"=w425) -> ()  [unwired: 2 in, 2 out]
      }
      frame True {
        w426 = T2."Enabled" ("Disabled")
        n154 = property on="Delay Value" class="DigNum (strict)"("DisabledEnum"=w426) -> ()  [unwired: 2 in, 2 out]
        n155 = property on="Add Delay" class="Bool (strict)"("DisabledEnum"=w426) -> ()  [unwired: 2 in, 2 out]
      }
    }
    n156 = Index Array(array=w161, index (row)=w266, index (col)=w266) -> (element=w265:variant)
    n157 = Index Array(array=w163) -> (element=w277:variant[])  [unwired: 2 in]
    n158 = Or(x=w322, y="stop") -> (x .or. y?=w318:bool)
    "stopping" <- w318
    n159 = local read "Auto Threshold"() -> (w220:bool)
    n160 = xnode "Database Variant To Data"("database variant"=w265, "type"=0.0) -> ("data"=w149:dbl)  [unwired: 1 in, 1 out]
    "Peletron (MV)" <- w149
    n161 = Equal To 0?(x=w149) -> (x = 0?=w150:bool)
    n162 = Index Array(array=w277, index #1=1 ("index"), index #2=2 ("index"), index #3=3 ("index"), index #4=4 ("index"), index #5=5 ("index"), index #6=6 ("index"), index #7=7 ("index"), index #8=8 ("index")) -> (element #1=w276:variant, element #2=w275:variant, element #3=w274:variant, element #4=w273:variant, element #5=w272:variant, element #6=w271:variant, element #7=w270:variant, element #8=w269:variant)
    n163 = case shown="True" w150 {
      tunnel: [w325 7600.0 ("Value")] -> w148
      tunnel: w149 -> [w325 _]
      frame False {
      }
      frame True {
      }
    }
    n164 = Or(x=w220, y=w222) -> (x .or. y?=w221:bool)
    n165 = case shown="True" w241 {
      frame False {
      }
      frame True {
        n166 = stacked-sequence {
          frame #0 {
            n167 = property on="Delay Ring" class="Ring (strict)"() -> ("StringsAndValues[]"=w430:T6)  [unwired: 2 in, 2 out]
            n168 = Bundle("Delay Name"="Delay Name", "Delay Value"="Delay Value") -> (w435:cluster{"Delay Name":string, "Delay Value":dbl})  [unwired: 1 in]
            n169 = Array Size(array=w430) -> (size(s)=w433:i32)
            n170 = for {
              tunnel: w430 -> [w440] mode=indexing
              tunnel: [w439] -> w429 mode=indexing
              n171 = Unbundle(w440) -> ("Value"=w439:dbl)  [unwired: 1 out]
            }
            n172 = Decrement(x=w433) -> (x-1=w432:i32)
            n173 = Search 1D Array(1D array=w429, element="Delay Value") -> (index of element=w437:i32)  [unwired: 1 in]
            n174 = Insert Into Array(array=w430, index=w432, new element=w435) -> (w434:T6)
            n175 = Equal?(x=w437, y=-1) -> (x = y?=w431:bool)
            n176 = case shown="True" w431 {
              tunnel: w434 -> [_ w449]
              frame False {
                n177 = One Button Dialog(message="Value Already Exists") -> ()  [unwired: 1 in, 1 out]
              }
              frame True {
                n178 = Array Size(array=w449) -> (size(s)=w451:i32)
                n179 = Decrement(x=w451) -> (x-1=w450:i32)
                n180 = call <userlib>:"Current VI's Path__ogtk.vi"() -> ("Current VI's Path (+ Relative)"=w455:path)  [unwired: 1 in]
                n181 = for {
                  N: w450 -> [_]
                  tunnel: w449 -> [w465] mode=indexing
                  tunnel: [w460] -> w452 mode=indexing
                  n182 = Unbundle(w465) -> ("String"=w461:string, "Value"=w464:dbl)
                  n183 = Format Into String(format string="%f", w464) -> (resulting string=w462:string)  [unwired: 2 in, 1 out]
                  n184 = Build Array(w461, w462) -> (w460:string[])
                }
                n185 = property on="Delay Ring" class="Ring (strict)"("StringsAndValues[]"=w449) -> ()  [unwired: 2 in, 2 out]
                n186 = Strip Path(path=w455) -> (stripped path=w443:path)  [unwired: 1 out]
                n187 = call-poly <userlib>:"Strip Path Extension__ogtk.vi"("path"=w443) -> ("extension"=w446:string)  [unwired: 1 out]
                n188 = Equal?(x="exe", y=w446) -> (x = y?=w444:bool)
                n189 = case shown="False" w444 {
                  tunnel: w443 -> [w457 w459]
                  tunnel: [w457 w458] -> w442
                  frame False {
                  }
                  frame True {
                    n190 = Strip Path(path=w459) -> (stripped path=w458:path)  [unwired: 1 out]
                  }
                }
                n191 = Array To Spreadsheet String(array=w452, 3:"%s" ("format string")) -> (spreadsheet string=w448:string)  [unwired: 1 in]
                n192 = Build Path(base path=w442, name or relative path="delay_ring.txt") -> (appended path=w453:path)
                n193 = call <vilib>:"Trim Whitespace.vi"("string"=w448) -> ("trimmed string"=w447:string)  [unwired: 1 in]
                n194 = Write to Text File(file (use dialog)=w453, text=w447) -> ()  [unwired: 2 in, 3 out]
              }
            }
          }
          frame #1 {
            n195 = property on="Add Delay" class="Bool (strict)"("Value"=FALSE ("Add Delay")) -> ()  [unwired: 2 in, 2 out]
          }
        }
      }
    }
    n196 = xnode "Read/Write Control"("FPGA VI Reference In"=w152, "error in"=w238, "One Shot"="One Shot Mode", "Reset One Shot"="Rearm Trigger") -> ("FPGA VI Reference Out"=w232:refnum<k20>, "error out"=w231:errorcluster)
    n197 = xnode "Database Variant To Data"("database variant"=w275, "type"=w268) -> ("data"=w201:dbl)  [unwired: 1 in, 1 out]
    n198 = xnode "Database Variant To Data"("database variant"=w276, "type"=w268) -> ("data"=w202:dbl)  [unwired: 1 in, 1 out]
    n199 = xnode "Database Variant To Data"("database variant"=w273, "type"=w268) -> ("data"=w200:dbl)  [unwired: 1 in, 1 out]
    n200 = xnode "Database Variant To Data"("database variant"=w274, "type"=w268) -> ("data"=w199:dbl)  [unwired: 1 in, 1 out]
    n201 = xnode "Database Variant To Data"("database variant"=w271, "type"=w268) -> ("data"=w198:dbl)  [unwired: 1 in, 1 out]
    n202 = xnode "Database Variant To Data"("database variant"=w272, "type"=w268) -> ("data"=w197:dbl)  [unwired: 1 in, 1 out]
    n203 = xnode "Database Variant To Data"("database variant"=w270, "type"=w267) -> ("data"=w260:i8)  [unwired: 1 in, 1 out]
    n204 = xnode "Database Variant To Data"("database variant"=w269, "type"=w267) -> ("data"=w259:i8)  [unwired: 1 in, 1 out]
    n205 = Build Array(w201, w202) -> (w263:dbl[])
    n206 = Build Array(w200, w199) -> (w262:dbl[])
    n207 = Build Array(w198, w197) -> (w261:dbl[])
    n208 = Equal To 0?(x="Delay Ring") -> (x = 0?=w196:bool)
    n209 = call "calc_variables.vi"("var2"=w259, "Peletron"=w148, "var1"=w260, "Mass"=w261, "Charge"=w262, "Velocity"=w263) -> ("Mass out"=w252:dbl[], "Charge out"=w255:dbl[], "Velocity out"=w258:dbl[])  [unwired: 3 in]
    n210 = xnode "Read/Write Control"("FPGA VI Reference In"=w232, "error in"=w231) -> ("Not Armed?"=w230:bool, "Del Not Armed?"=w190:bool)  [unwired: 2 out]
    n211 = local read "Delay Value"() -> (w195:dbl)
    n212 = property on="Rearm Trigger" class="Bool (strict)"(error in=w231, "Value"=FALSE ("Rearm Trigger")) -> ()  [unwired: 1 in, 2 out]
    n213 = Divide(x="Delay Ring", y=0.93) -> (x/y=w228:dbl)
    n214 = Select(t=w195, s=w196, f=w228) -> (s? t:f=w227:dbl)
    n215 = Not(x=w230) -> (.not. x?=→"Armed":bool)
    n216 = Not(x=w190) -> (.not. x?=→"Del Armed":bool)
    n217 = And(x=w196, y=w191) -> (x .and. y?=w192:bool)
    n218 = case shown="True" w192 {
      selector: w192 -> [w419 _]
      tunnel: w195 -> [_ w421]
      tunnel: [w419 w420] -> w193
      frame False {
      }
      frame True {
        n219 = call-poly <userlib>:"Data Changed__ogtk.vi"("DBL"=w421) -> ("Changed"=w420:bool)
      }
    }
    n220 = To Fixed-Point(number=w227) -> (fixed-point=w240:fxp<+,16,7>)  [unwired: 1 in]
    n221 = Index Array(array=w255, index #1=0 ("index"), index #2=1 ("index")) -> (element #1=w247:dbl, element #2=w246:dbl)
    "High Charge Limit (fC)" <- w246
    "Low Charge Limit (fC)" <- w247
    n222 = Index Array(array=w258, index #1=0 ("index"), index #2=1 ("index")) -> (element #1=w249:dbl, element #2=w248:dbl)
    "High Velocity" <- w248
    "Low Velocity" <- w249
    n223 = Index Array(array=w252, index #1=0 ("index"), index #2=1 ("index")) -> (element #1=w245:dbl, element #2=w244:dbl)
    "Low Mass (kg)" <- w245
    "High Mass (kg)" <- w244
    n224 = Bundle("Numeric"=w249, "Numeric"=w248, "Numeric"=w247, "Numeric"=w246, "Numeric"=w245, "Numeric"=w244, "Sensitivity"=w151, 26666666.6, "Value"=w148, w240, w191) -> (w295:T7)  [unwired: 1 in]
    n225 = call "process_limits.vi"("old output cluster"=w302, "Input cluster"=w295) -> ("Update FPGA"=w243:bool, "output cluster"=w303:T8)  [unwired: 8 in]
    n226 = Unbundle By Name(w303) -> ("Low Velocity Count"=w291:i32, "High Velocity Count"=w290:i32, "Low Charge Limit (ADC ticks)"=w288:i16, "High Charge Limit (ADC ticks)"=w289:i16, "Low Mass (ADC*cycle^2)"=w293:i64, "High Mass (ADC*cycle^2)"=w294:i64, "Mult"=w239:fxp<+,16,7>)
    "Low velocity count" <- w291
    "High velocity count" <- w290
    "High Charge Limit" <- w289
    "Low Charge Limit" <- w288
    "High Mass Limit" <- w294
    "Low Mass Limit" <- w293
    n227 = Or(x=w243, y=w221) -> (x .or. y?=w226:bool)
    n228 = Or(x="Raise Threshold", y="Lower Threshold") -> (x .or. y?=w203:bool)
    n229 = Or(x=w203, y=w226) -> (x .or. y?=w204:bool)
    n230 = Build Array("Filter1 Threshold", "Filter2 Threshold", "Filter3 Threshold", "Filter4 Threshold", "Filter5 Threshold", "Filter6 Threshold", "Filter7 Threshold") -> (w171:i32[])
    n231 = Or(x=w204, y=w193) -> (x .or. y?=w194:bool)
    "Updating FPGA" <- w194
    n232 = Build Array("Threshold 1", "Threshold 2", "Threshold 3", "Threshold 4", "Threshold 5", "Threshold 6", "Threshold 7") -> (w178:bool[])
    n233 = Initialize Array("Update All", 7 ("dimension size")) -> (w179:bool[])
    n234 = Or(x=w179, y=w178) -> (x .or. y?=w172:bool[])
    n235 = Initialize Array("Update By", 7 ("dimension size")) -> (w173:i32[])
    n236 = case shown="True" "Raise Threshold" {
      tunnel: w171 -> [_ w395]
      tunnel: w172 -> [_ w396]
      tunnel: w173 -> [_ w394]
      frame False {
      }
      frame True {
        n237 = Index Array(array=w396) -> (element #1=w417:bool, element #2=w416:bool, element #3=w415:bool, element #4=w414:bool, element #5=w413:bool, element #6=w412:bool, element #7=w411:bool)  [unwired: 7 in]
        n238 = Subtract(x=w395, y=w394) -> (x-y=w418:i32[])
        n239 = Select(t=w418, s=w417, f=w395) -> (s? t:f=w410:i32[])
        n240 = Select(t=w418, s=w416, f=w395) -> (s? t:f=w406:i32[])
        n241 = Select(t=w418, s=w412, f=w395) -> (s? t:f=w399:i32[])
        n242 = Select(t=w418, s=w414, f=w395) -> (s? t:f=w403:i32[])
        n243 = Select(t=w418, s=w413, f=w395) -> (s? t:f=w401:i32[])
        n244 = Select(t=w418, s=w411, f=w395) -> (s? t:f=w397:i32[])
        n245 = Select(t=w418, s=w415, f=w395) -> (s? t:f=w405:i32[])
        n246 = Index Array(array=w406, index=1) -> (element=w391:i32)
        n247 = Index Array(array=w410, index=0) -> (element=w392:i32)
        n248 = Index Array(array=w397, index=6) -> (element=w386:i32)
        n249 = Index Array(array=w401, index=4) -> (element=w388:i32)
        n250 = Index Array(array=w405, index=2) -> (element=w390:i32)
        n251 = Index Array(array=w403, index=3) -> (element=w389:i32)
        n252 = Index Array(array=w399, index=5) -> (element=w387:i32)
        n253 = local write "Filter1 Threshold"(w392) -> ()
        n254 = local write "Filter6 Threshold"(w387) -> ()
        n255 = local write "Filter5 Threshold"(w388) -> ()
        n256 = local write "Filter7 Threshold"(w386) -> ()
        n257 = local write "Filter3 Threshold"(w390) -> ()
        n258 = local write "Filter2 Threshold"(w391) -> ()
        n259 = local write "Filter4 Threshold"(w389) -> ()
        n260 = local write "Raise Threshold"(FALSE ("Raise Threshold")) -> ()
      }
    }
    n261 = case shown="False" "Lower Threshold" {
      tunnel: w171 -> [w351 w375]
      tunnel: w173 -> [_ w385]
      tunnel: w172 -> [_ w384]
      tunnel: [w351 w352] -> w170
      frame False {
      }
      frame True {
        n262 = Index Array(array=w384) -> (element #1=w382:bool, element #2=w381:bool, element #3=w380:bool, element #4=w379:bool, element #5=w378:bool, element #6=w377:bool, element #7=w376:bool)  [unwired: 7 in]
        n263 = Add(x=w375, y=w385) -> (x+y=w383:i32[])
        n264 = Select(t=w383, s=w382, f=w375) -> (s? t:f=w374:i32[])
        n265 = Select(t=w383, s=w381, f=w375) -> (s? t:f=w370:i32[])
        n266 = Select(t=w383, s=w377, f=w375) -> (s? t:f=w363:i32[])
        n267 = Select(t=w383, s=w379, f=w375) -> (s? t:f=w367:i32[])
        n268 = Select(t=w383, s=w378, f=w375) -> (s? t:f=w365:i32[])
        n269 = Select(t=w383, s=w376, f=w375) -> (s? t:f=w361:i32[])
        n270 = Select(t=w383, s=w380, f=w375) -> (s? t:f=w369:i32[])
        n271 = Index Array(array=w370, index=1) -> (element=w358:i32)
        n272 = Index Array(array=w374, index=0) -> (element=w359:i32)
        n273 = Index Array(array=w361, index=6) -> (element=w353:i32)
        n274 = Index Array(array=w365, index=4) -> (element=w355:i32)
        n275 = Index Array(array=w369, index=2) -> (element=w357:i32)
        n276 = Index Array(array=w367, index=3) -> (element=w356:i32)
        n277 = Index Array(array=w363, index=5) -> (element=w354:i32)
        n278 = local write "Filter4 Threshold"(w356) -> ()
        n279 = local write "Filter6 Threshold"(w354) -> ()
        n280 = local write "Filter3 Threshold"(w357) -> ()
        n281 = local write "Filter5 Threshold"(w355) -> ()
        n282 = local write "Filter7 Threshold"(w353) -> ()
        n283 = local write "Filter2 Threshold"(w358) -> ()
        n284 = local write "Filter1 Threshold"(w359) -> ()
        n285 = local write "Lower Threshold"(FALSE ("Lower Threshold")) -> ()
        n286 = Build Array(w359, w358, w357, w356, w355, w354, w353) -> (w352:i32[])
      }
    }
    n287 = Index Array(array=w170) -> (element #1=w217:i32, element #2=w215:i32, element #3=w213:i32, element #4=w211:i32, element #5=w209:i32, element #6=w207:i32, element #7=w205:i32)  [unwired: 7 in]
    n288 = case shown="True" w194 {
      tunnel: w152 -> [w468 w496]
      tunnel: w238 -> [w469 w495]
      tunnel: [w468 w494] -> w320
      tunnel: [w469 w493] -> w319
      tunnel: w217 -> [_ w475]
      tunnel: w215 -> [_ w476]
      tunnel: w213 -> [_ w474]
      tunnel: w211 -> [_ w473]
      tunnel: w209 -> [_ w472]
      tunnel: w207 -> [_ w471]
      tunnel: w205 -> [_ w470]
      tunnel: [w467 w479] -> w300
      tunnel: w294 -> [_ w485]
      tunnel: w293 -> [_ w484]
      tunnel: w291 -> [_ w483]
      tunnel: w290 -> [_ w482]
      tunnel: w289 -> [_ w481]
      tunnel: w288 -> [_ w480]
      tunnel: w301 -> [w467 _]
      tunnel: w239 -> [_ w477]
      frame False {
      }
      frame True {
        n289 = xnode "Read/Write Control"("FPGA VI Reference In"=w496, "error in"=w495, "Low Velocity Count"=w483, "High Velocity Count"=w482, "Filter 1 threshold"=w475, "Filter 2 threshold"=w476, "Filter 3 threshold"=w474, "Filter 4 threshold"=w473, "Filter 5 threshold"=w472, "Filter 6 threshold"=w471, "Filter 7 threshold"=w470, "High Charge Limit"=w481, "Low Charge Limit"=w480, "High Mass Limit"=w485, "Low Mass Limit"=w484, "Mult1"=w477) -> ("FPGA VI Reference Out"=w494:refnum<k20>, "error out"=w493:errorcluster, "Filter 1 Detector 3 Correlation"=w492:i32, "Filter 2 Detector 3 Correlation"=w491:i32, "Filter 3 Detector 3 Correlation"=w490:i32, "Filter 4 Detector 3 Correlation"=w489:i32, "Filter 5 Detector 3 Correlation"=w488:i32, "Filter 6 Detector 3 Correlation"=w487:i32, "Filter 7 Detector 3 Correlation"=w486:i32)
        n290 = Get Date/Time In Seconds() -> (seconds since 1Jan1904=→"Last Update:":timestamp)
        n291 = Bundle("Filter 1 Detector 3 Correlation"=w492, "Filter 2 Detector 3 Correlation"=w491, "Filter 3 Detector 3 Correlation"=w490, "Filter 4 Detector 3 Correlation"=w489, "Filter 5 Detector 3 Correlation"=w488, "Filter 6 Detector 3 Correlation"=w487, "Filter 7 Detector 3 Correlation"=w486) -> (w479:T9)  [unwired: 1 in]
      }
    }
    n292 = call "filter_peaks.vi"("Correlation cluster"=w300, "Filter peak cluster"=w296, "Zero out"="Zero Peak Values", "Run Mode"="Run Mode") -> ("Blinking"=w287:bool, "status"=w292:T2, "Filter peak output"=w297:T5)  [unwired: 5 in]
    n293 = shared-variable "My Computer\\Network Shared Variables.lvlib\\FPGA Trigger"() -> ()  [unwired: 1 in, 2 out]
    n294 = Unbundle By Name(w297) -> ("Filter 1 Peak"=w317:i32, "Filter 2 Peak"=w316:i32, "Filter 3 Peak"=w315:i32, "Filter 4 Peak"=w314:i32, "Filter 5 Peak"=w313:i32, "Filter 6 Peak"=w312:i32, "Filter 7 Peak"=w311:i32)
    "Filter 1 Peak" <- w317
    "Filter 2 Peak" <- w316
    "Filter 3 Peak" <- w315
    "Filter 4 Peak" <- w314
    "Filter 5 Peak" <- w313
    "Filter 6 Peak" <- w312
    "Filter 7 Peak" <- w311
    n295 = property on="Filter 3 Peak" class="DigNum (strict)"("DisabledEnum"=w292, "Blinking"=w287) -> ()  [unwired: 2 in, 2 out]
    n296 = property on="Filter 4 Peak" class="DigNum (strict)"("DisabledEnum"=w292, "Blinking"=w287) -> ()  [unwired: 2 in, 2 out]
    n297 = property on="Filter 7 Peak" class="DigNum (strict)"("DisabledEnum"=w292, "Blinking"=w287) -> ()  [unwired: 2 in, 2 out]
    n298 = property on="Filter 5 Peak" class="DigNum (strict)"("DisabledEnum"=w292, "Blinking"=w287) -> ()  [unwired: 2 in, 2 out]
    n299 = property on="Filter 6 Peak" class="DigNum (strict)"("DisabledEnum"=w292, "Blinking"=w287) -> ()  [unwired: 2 in, 2 out]
    n300 = property on="Filter 2 Peak" class="DigNum (strict)"("DisabledEnum"=w292, "Blinking"=w287) -> ()  [unwired: 2 in, 2 out]
    n301 = property on="Filter 1 Peak" class="DigNum (strict)"("DisabledEnum"=w292, "Blinking"=w287) -> ()  [unwired: 2 in, 2 out]
    n302 = local read "Update Threshold"() -> (w153:bool)
    n303 = case shown="True" w153 {
      frame False {
      }
      frame True {
        n304 = local write "Update Threshold"(FALSE ("Update Threshold")) -> ()
      }
    }
    n305 = Or(x=w220, y=w153) -> (x .or. y?=w219:bool)
    "Sensitivity" <- w151
  }
  n306 = while {
    stop <- w786 stop-if-true
    n307 = case shown="True" "Rate Limiting" {
      frame False {
        n308 = property on="Rearm Trigger" class="Bool (strict)"("DisabledEnum"=T2."Enabled" ("Disabled")) -> ()  [unwired: 2 in, 2 out]
        n309 = property on="One Shot Mode" class="Bool (strict)"("DisabledEnum"=T2."Enabled" ("Disabled")) -> ()  [unwired: 2 in, 2 out]
      }
      frame True {
        n310 = local read "Armed"() -> (w790:bool)
        n311 = Get Date/Time In Seconds() -> (seconds since 1Jan1904=w789:timestamp)
        n312 = property on="Rearm Trigger" class="Bool (strict)"("DisabledEnum"=T2."Disabled and Grayed Out" ("Disabled")) -> ()  [unwired: 2 in, 2 out]
        n313 = case shown="False" w790 {
          tunnel: [w797 FALSE] -> w794
          tunnel: w789 -> [w796 _]
          frame False {
            n314 = flat-sequence {
              tunnel: w796 -> [w798]
              tunnel: [w798] -> w795
              tunnel: [TRUE] -> w797
              tunnel: w795 -> [w804]
              frame #0 {
                n315 = Multiply(x="Min. Time\nBetween Shots (s)", y=1000.0) -> (x*y=w801:dbl)
                n316 = Round Toward +Infinity(x=w801) -> (ceil(x): smallest int >= x=w799:dbl)
                n317 = Wait (ms)(milliseconds to wait=w799) -> ()  [unwired: 1 out]
              }
              frame #1 {
                n318 = Get Date/Time In Seconds() -> (seconds since 1Jan1904=w805:timestamp)
                n319 = Subtract(x=w805, y=w804) -> (x-y=→"Time Betwee Shots":dbl)
              }
            }
          }
          frame True {
          }
        }
        n320 = property on="One Shot Mode" class="Bool (strict)"("DisabledEnum"=T2."Disabled and Grayed Out" ("Disabled"), "Value"=TRUE ("One Shot Mode")) -> ()  [unwired: 2 in, 2 out]
        n321 = local write "Rearm Trigger"(w794) -> ()
      }
    }
    n322 = property on="stopping" class="Bool (strict)"() -> ("Value"=w786:bool)  [unwired: 2 in, 2 out]
  }
  n323 = call "connect out.vi"("error in (no error)"=w41, "connection reference"=w43) -> ()  [unwired: 9 in, 1 out]
  n324 = xnode "Close FPGA VI Reference"("FPGA VI Reference In"=w66, "error in"=w65) -> ("error out"=w68:errorcluster)
  n325 = call <vilib>:"General Error Handler.vi"("error in (no error)"=w68) -> ()  [unwired: 10 in, 5 out]
